vi "Scope_5160.vi"() -> ()   [LabVIEW 2013]
uses:
  <vilib>/rvi/interface/nirviReadWriteControl/nirviReadWriteControl.xnode
  <vilib>/rvi/errors/niLvFpgaAdjustHostInterfaceError.vi
  <vilib>/rvi/interface/nirviCloseFPGA/nirviCloseFPGA.xnode
  FPGA/DataMode.ctl
  NiFpgaLv.dll
  <vilib>/Utility/error.llb/Error Cluster From Error Code.vi
  <vilib>/rvi/interface/Simulation/niFpgaSimulationCallBeginRW.vi
  Host/Utilities/Ticker/Ticker.lvclass
  Host/Scope/controls/ScopeMode.ctl
  <vilib>/rvi/interface/nirviOpenFPGA/nirviOpenFPGA.xnode
  Host/Config/5160FPGAref.ctl
  Host/Scope/P2P streaming/trigger_source.ctl
  <vilib>/FPGAPlugInAG/Dynamic/niLvFpga_Close_Dynamic.vi
  FPGA Bitfiles/mixer_FPGATarget_FPGAmain5160_6pHC8ZmJ734.lvbitx
  <vilib>/FPGAPlugInAG/PXIe-7975R/niLvFpga_Open_PXIe-7975R.vi
  <vilib>/rvi/interface/common/dynamic/niFpgaDynamicAddResources.vi
  Host/Config/FPGAref.ctl
  <vilib>/userdefined/High Color/nirio_resource_hc.ctl
  <vilib>/Analysis/4window.llb/windowTd.ctl
  <vilib>/Analysis/NI_AALPro.lvlib
  Host/Scope/controls/power_spectrum_unit.ctl
panel:
  out "stop 2":bool
  out "num data 2nd loop":u32
  out "timeout counter":i32
  out "num read":u32
  out "num to clock fifo":u32
  out "error out":errorcluster
  out "P2P overflow":bool
  in  "Trigger":T1
  in  "Zoom freq X":bool
  in  "Zoom freq Y":bool
  in  "Zoom time Y":bool
  in  "Zoom time X":bool
  in  "Ch3":bool
  in  "Ch2":bool
  in  "Ch3 Q":bool
  in  "Ch3 I":bool
  in  "Ch2 Q":bool
  in  "Ch2 I":bool
  in  "input impedance":u32(ring) caption="Input Impedance" items=["1 mega ohm"=0, "50 ohms"=2]
  in  "SCOPE Resource":refnum<k15>="Dev1" caption="NI-Scope Resource"
  in  "Unit":T2
  in  "Window":T3=1 items=["Rectangle"=0, "Hanning"=1, "Hamming"=2, "Blackman-Harris"=3, "Exact Blackman"=4, "Blackman"=5, "Flat Top"=6, "4 Term B-Harris "=7, "7 Term B-Harris"=8, "Low Sidelobe"=9, "Blackman Nuttall"=11, "Triangle"=30, "Bartlett-Hanning"=31, "Bohman"=32, "Parzen"=33, "Welch"=34, "Kaiser"=60, "Dolph-Chebyshev"=61, "Gaussian"=62]
  in  "Samples per record":u32
  in  "Phase offset (deg)":dbl
  in  "Fequency [MHz]":dbl
  in  "Mode":T4
  in  "Mixer freq [MHz]":dbl
  in  "Ch1":bool
  in  "Ch0":bool
  out "freqdata":cluster{"f0":dbl, "df":dbl, "magnitude":dbl[]}[](graph)
  out "Timedata":i16[][](graph)
  in  "Rumode":bool
  in  "Singleshot":bool
  in  "Ch1 Q":bool
  in  "Ch1 I":bool
  in  "Ch0 Q":bool
  in  "Ch0 I":bool
  out "error IO":errorcluster
  in  "stop":bool
  in  "resource name":T5="RIO0"
  out "Clocking Option Configured?":bool
  out "Configured?":bool
  # "FPGA setup"
  # "Auto Zoom"
  # "Auto Zoom"
  # "FFT"
  # "Simulated data"
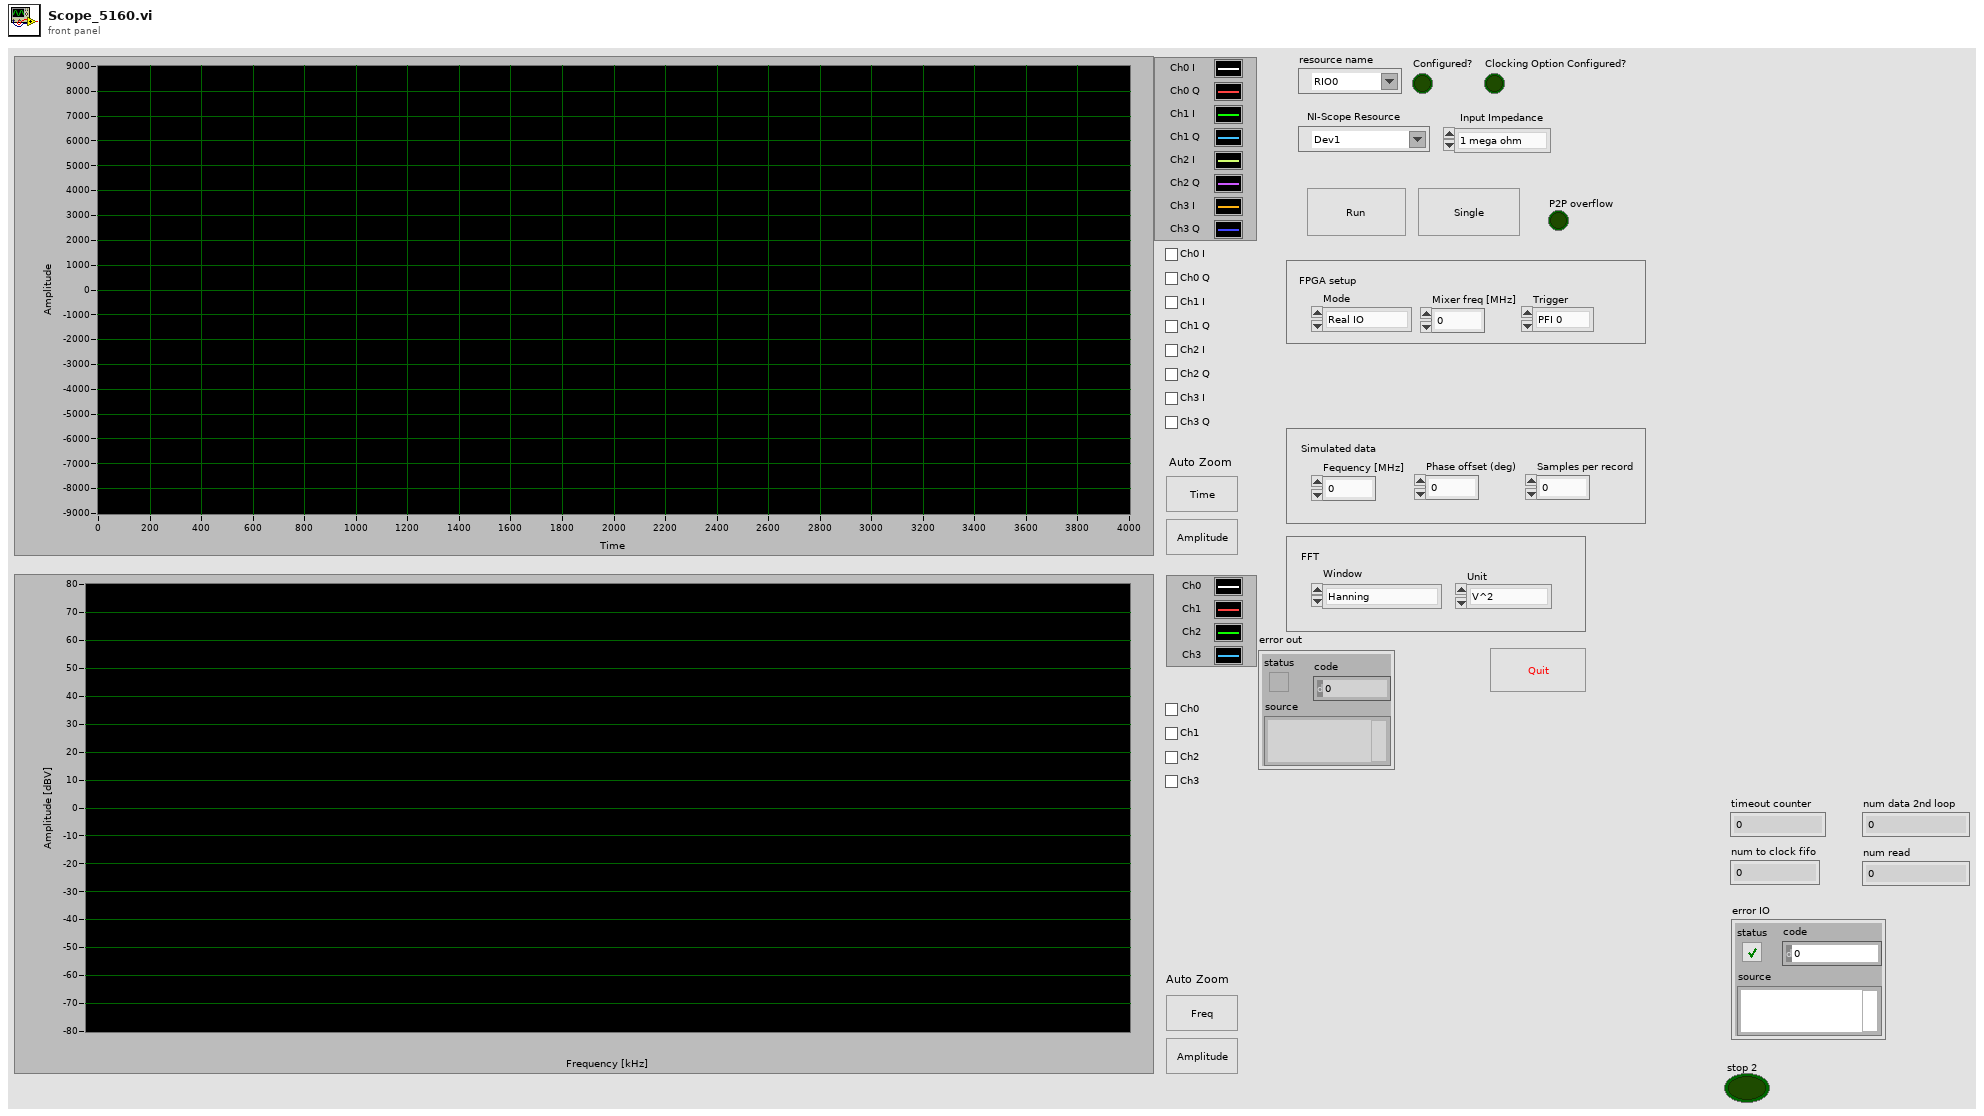
[diagram p1: front panel]
types:
  T1 = typedef "trigger_source.ctl" = enum16{"PFI 0", "PFI 1", "Software"}
  T2 = typedef "power_spectrum_unit.ctl" = enum16{"V^2", "V", "dBV"}
  T3 = typedef "NI_AALPro.lvlib/windowTd.ctl" = u32
  T4 = typedef "DataMode.ctl" = enum16{"Real IO", "Simulated"}
  T5 = typedef "nirio_resource_hc.ctl" = tag
  T6 = enum8{"Internal Clock PLL Off", "Internal Clock PLL On (REF IN)", "External Clock (CLK_IN)", "Internal Clock PLL On (IoModSyncClk)"}
  T7 = typedef "FPGAref.ctl" = refnum<k20>
  T8 = typedef "scope_params.ctl" = cluster{"scope mode":T9, "ticker":refnum<class "Ticker.lvclass">, "samples per simulated":u32, "FPGA ref":T7, "P2P params":T10, "data mode":T4}
  T9 = typedef "ScopeMode.ctl" = enum16{"Stopped", "Single", "Running"}
  T10 = typedef "P2P params.ctl" = cluster{"instrument handle":refnum<k15>, "stream session":refnum<k20>, "scale":cluster{"offset":dbl, "gain":dbl, "reserved 1":dbl, "reserved 2":dbl}, "actual sample rate":dbl, "Trigger":T1, "SCOPE Resource":refnum<k15>, "input impedance":u32}
  T11 = typedef "5160FPGAref.ctl" = refnum<k20>
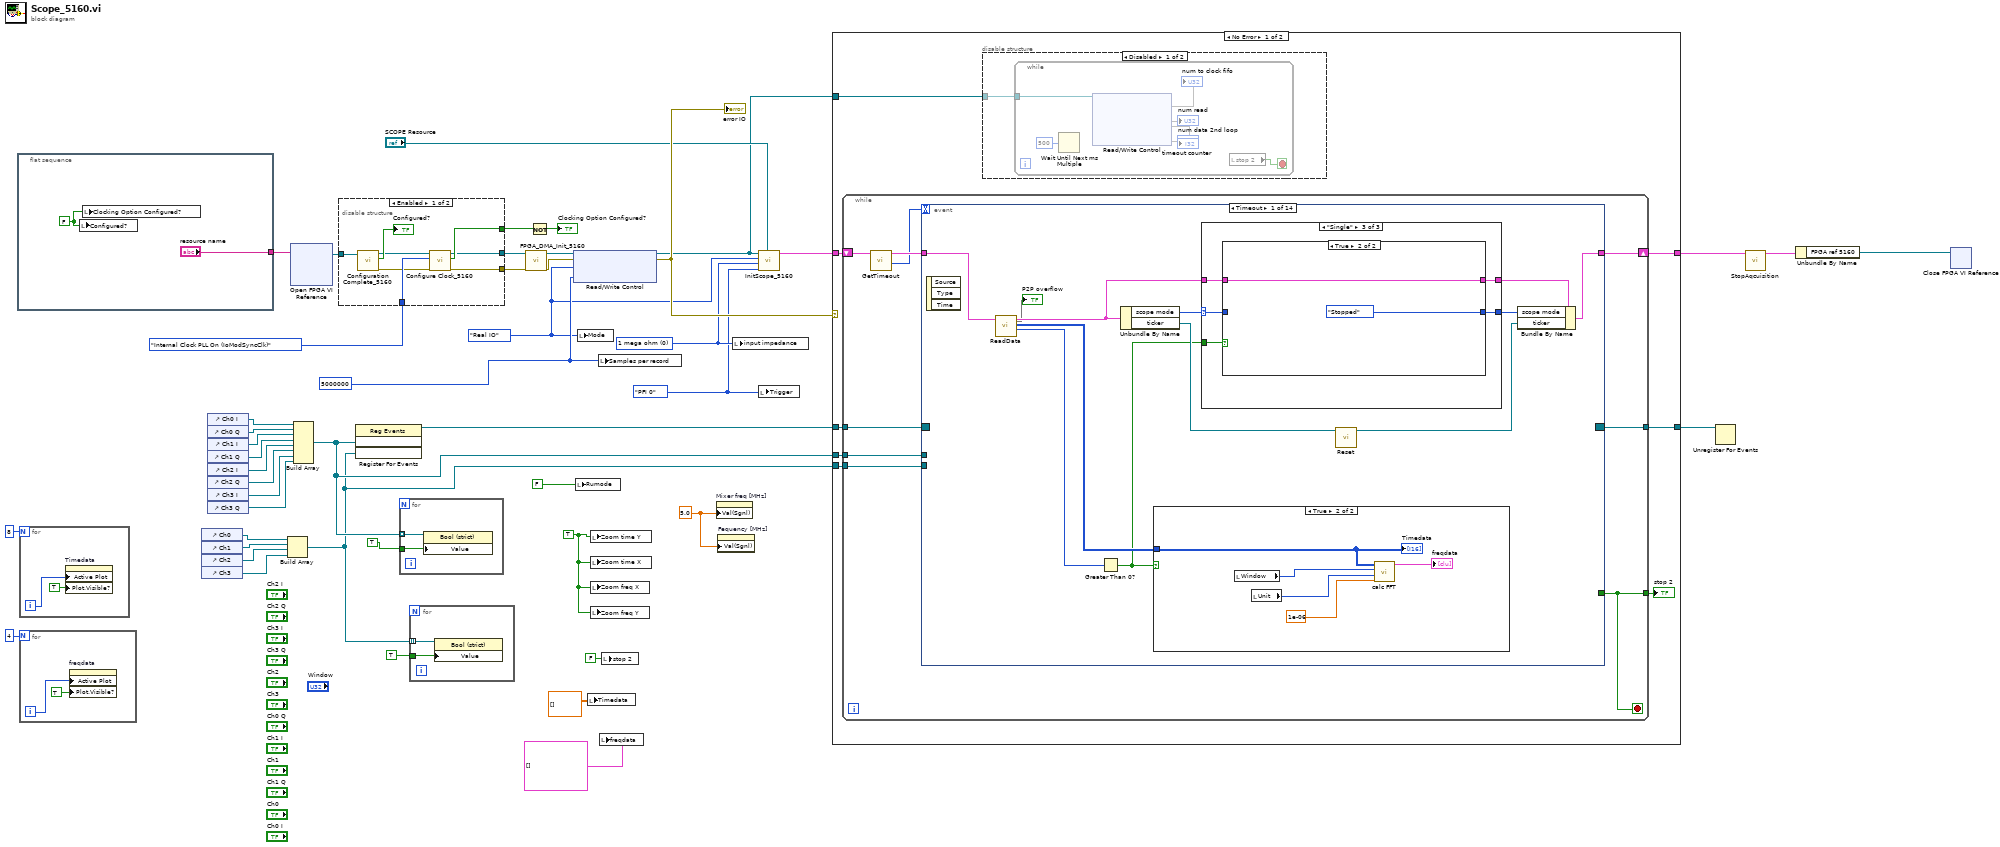
[diagram p0: block diagram]
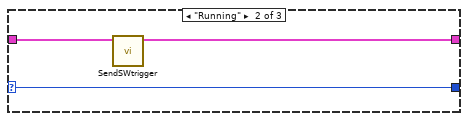
[diagram p6: hidden frame]
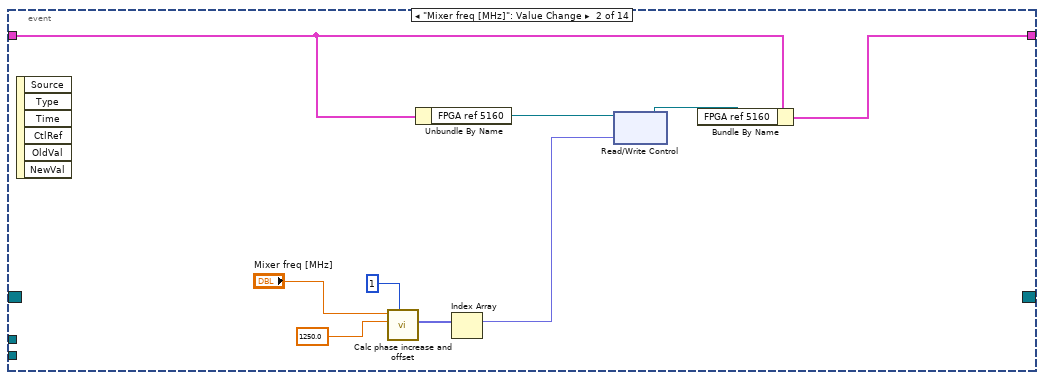
[diagram p8: hidden frame]
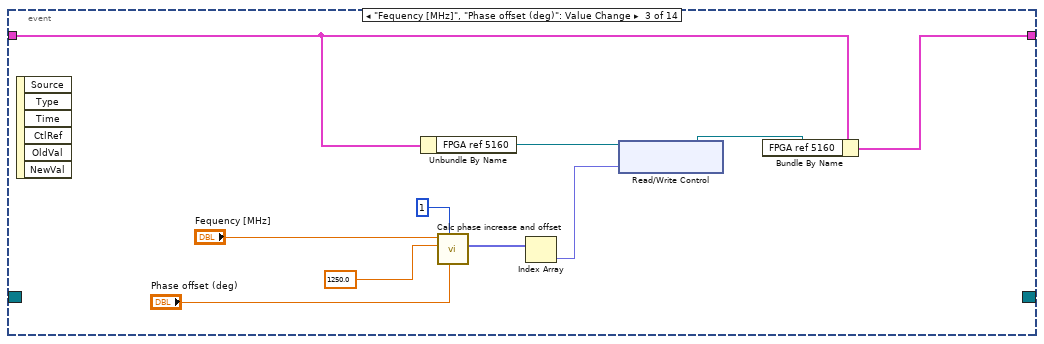
[diagram p9: hidden frame]
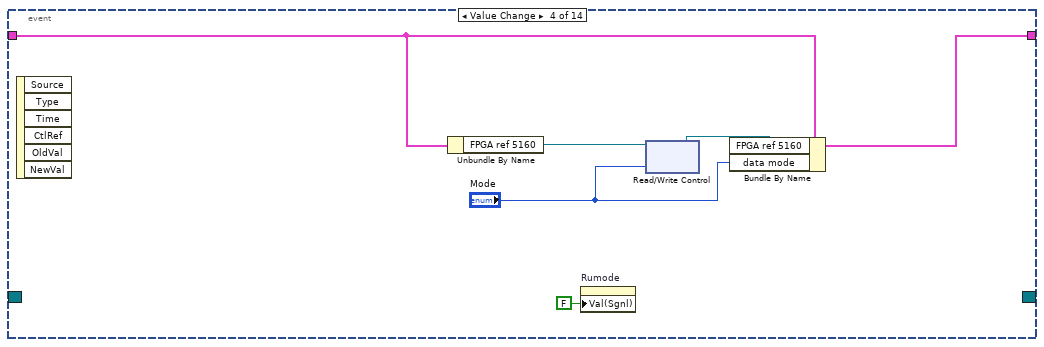
[diagram p10: hidden frame]
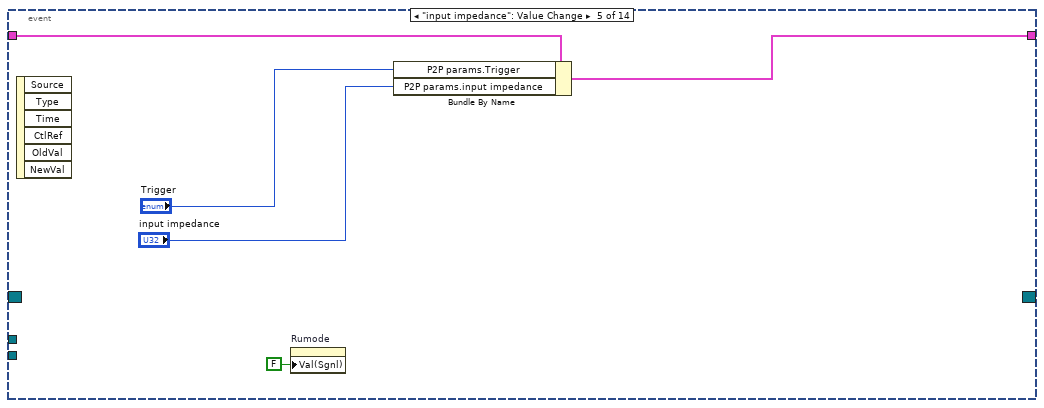
[diagram p11: hidden frame]
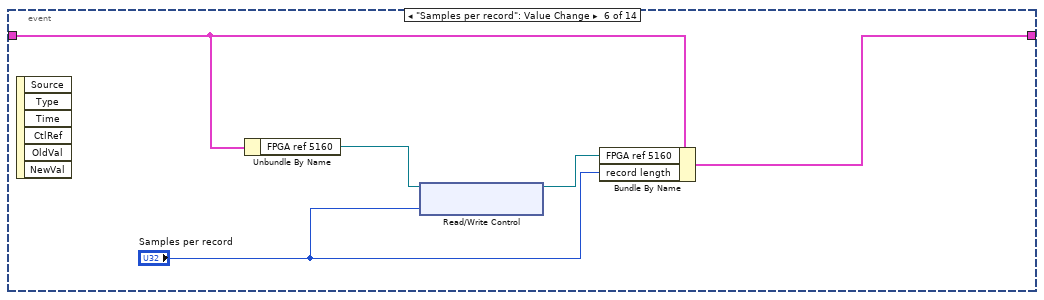
[diagram p12: hidden frame]
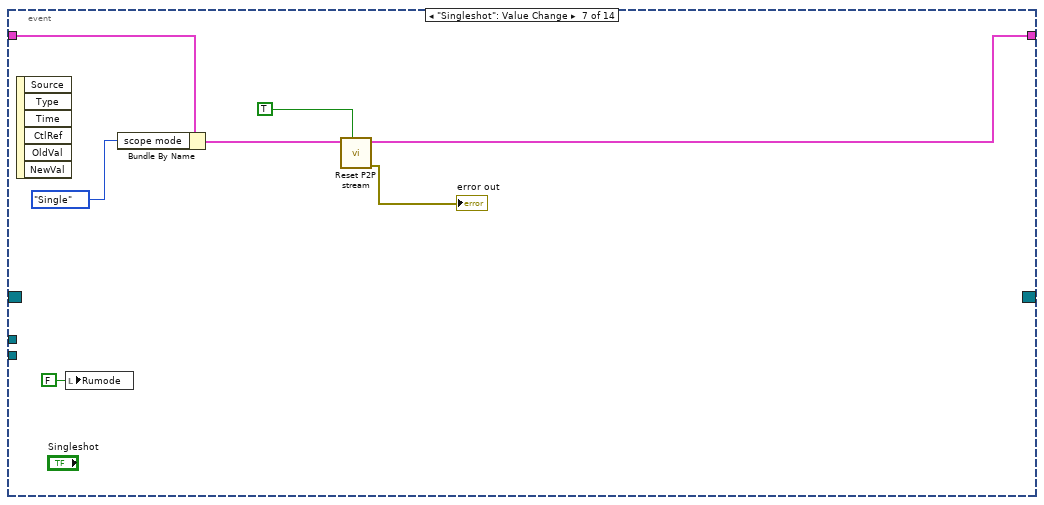
[diagram p13: hidden frame]
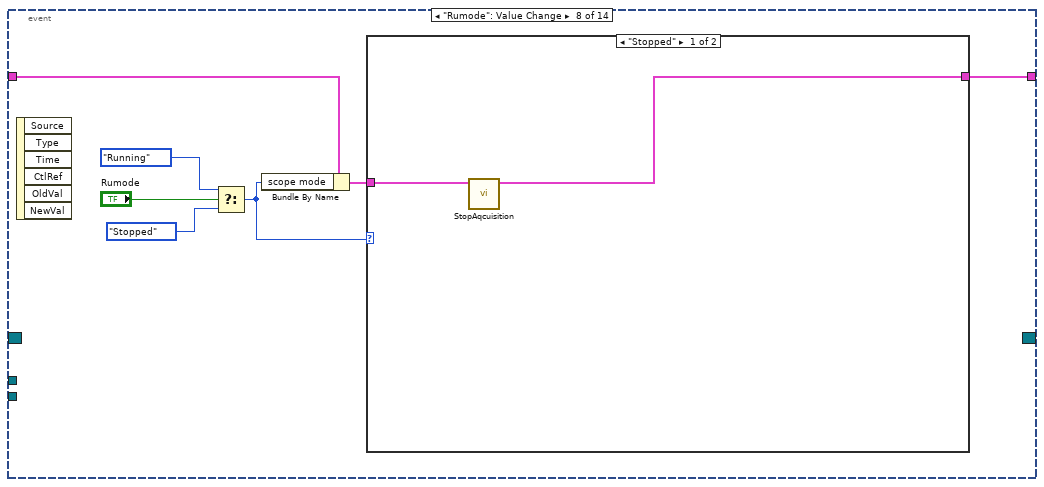
[diagram p14: hidden frame]
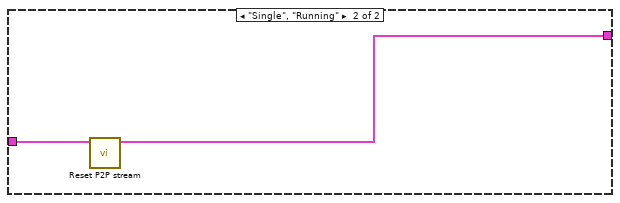
[diagram p15: hidden frame]
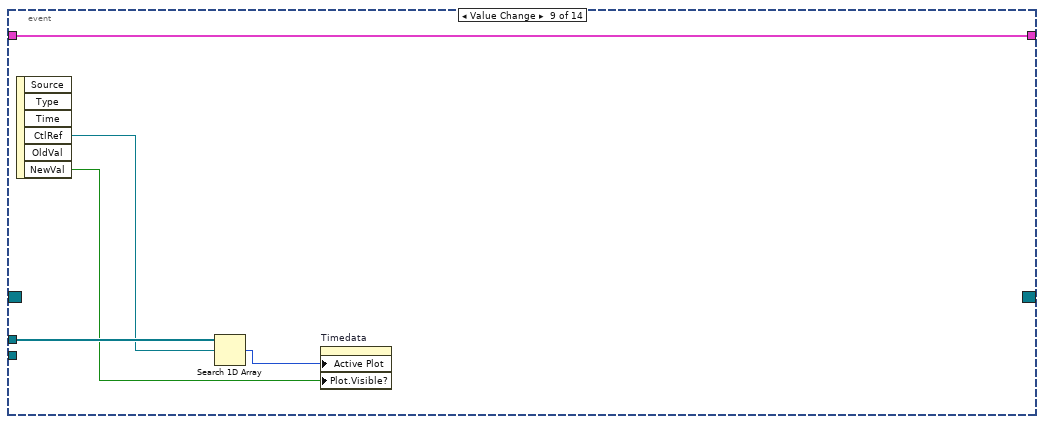
[diagram p16: hidden frame]
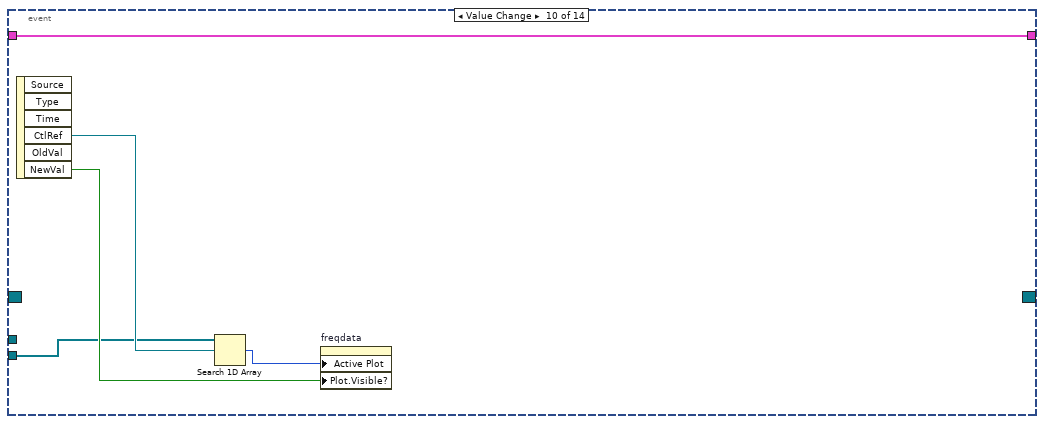
[diagram p17: hidden frame]
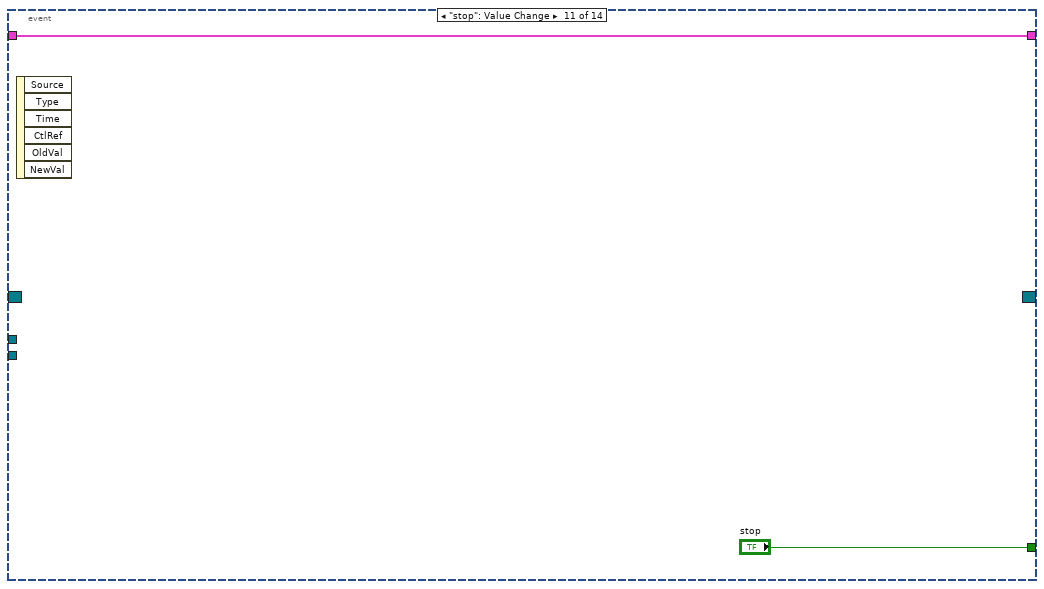
[diagram p18: hidden frame]
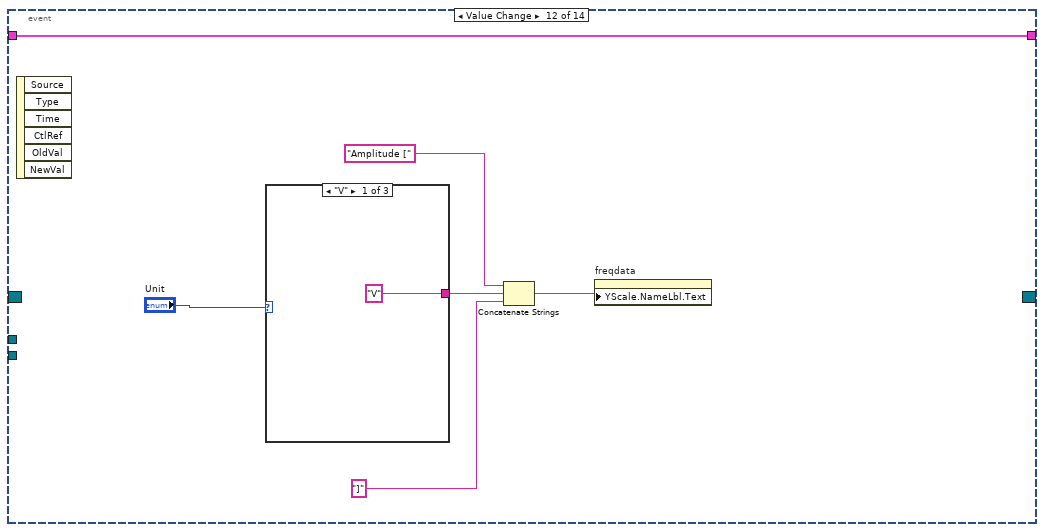
[diagram p19: hidden frame]
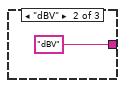
[diagram p20: hidden frame]
diagram:
  w4 = u32 0 items=["1 mega ohm"=0, "50 ohms"=2] ("input impedance")
  w3 = trigger_source."PFI 0" ("Trigger")
  w12 = TRUE ("Rumode")
  w5 = DataMode."Real IO" ("Mode")
  w7 = u32 5000000 ("Samples to aqcuire")
  w41 = 5.0 ("Mixer requency [MHz]")
  n1 = flat-sequence {
    tunnel: ["resource name"] -> w13
    frame #0 {
      w47 = FALSE ("Trigger Acquisition")
      n2 = local write "Configured?"(w47) -> ()
      n3 = local write "Clocking Option Configured?"(w47) -> ()
    }
  }
  n4 = for {
    N: 8 -> [_]
    i -> [w50]
    n5 = property on="Timedata" class="WFGraph (strict)"("Active Plot"=w50, "Plot.Visible?"=TRUE ("Plot.Visible")) -> ()  [unwired: 2 in, 2 out]
  }
  n6 = for {
    N: 4 -> [_]
    i -> [w51]
    n7 = property on="freqdata" class="WFGraph (strict)"("Active Plot"=w51, "Plot.Visible?"=TRUE ("Plot.Visible")) -> ()  [unwired: 2 in, 2 out]
  }
  n8 = control-ref of="Ch0"() -> (w26:refnum<vi>)
  n9 = control-ref of="Ch1"() -> (w25:refnum<vi>)
  n10 = control-ref of="Ch2"() -> (w24:refnum<vi>)
  n11 = control-ref of="Ch3"() -> (w23:refnum<vi>)
  n12 = control-ref of="Ch0 I"() -> (w37:refnum<vi>)
  n13 = control-ref of="Ch0 Q"() -> (w36:refnum<vi>)
  n14 = control-ref of="Ch1 I"() -> (w35:refnum<vi>)
  n15 = control-ref of="Ch1 Q"() -> (w34:refnum<vi>)
  n16 = control-ref of="Ch2 I"() -> (w33:refnum<vi>)
  n17 = control-ref of="Ch2 Q"() -> (w32:refnum<vi>)
  n18 = control-ref of="Ch3 I"() -> (w31:refnum<vi>)
  n19 = control-ref of="Ch3 Q"() -> (w30:refnum<vi>)
  n20 = Build Array(w26, w25, w24, w23) -> (w20:refnum<vi>[])
  n21 = xnode "Open FPGA VI Reference"("resource name"=w13) -> ("FPGA VI Reference Out"=w10:refnum<k20>)  [unwired: 1 in, 1 out]
  n22 = Build Array(w37, w36, w35, w34, w33, w32, w31, w30) -> (w21:refnum<vi>[])
  n23 = disable-structure shown="Enabled" {
    disable-tunnel: [w59 _] -> w18
    disable-tunnel: T6."Internal Clock PLL On (IoModSyncClk)" ("Clock Source") -> [w58 _]
    disable-tunnel: [w56 _] -> w15
    disable-tunnel: [w55 w61] -> w11
    disable-tunnel: w10 -> [w54 w61]
    frame Enabled {
      n24 = call "Configuration Complete_5160.vi"("FPGA VI Reference"=w54) -> ("error out"=w57:errorcluster, "Configured?"=→"Configured?":bool, "FPGA VI Reference out"=w53:refnum<k20>)  [unwired: 8 in]
      n25 = call "Configure Clock_5160.vi"("error in"=w57, "Clock Source"=w58, "FPGA VI Reference in"=w53) -> ("error out"=w56:errorcluster, "Configuration Error"=w59:bool, "FPGA VI Reference Out"=w55:refnum<k20>)  [unwired: 6 in]
    }
    frame Disabled {
    }
  }
  n26 = register-events(w21, w20) -> (reference out=w29:refnum<event-registration>)  [unwired: 2 in, 1 out]
  n27 = for {
    tunnel: w21 -> [w63] mode=indexing
    tunnel: TRUE ("Rumode") -> [w62]
    n28 = property class="Bool (strict)"(reference=w63, "Value"=w62) -> ()  [unwired: 1 in, 2 out]
  }
  n29 = for {
    tunnel: w20 -> [w65] mode=indexing
    tunnel: TRUE ("Rumode") -> [w64]
    n30 = property class="Bool (strict)"(reference=w65, "Value"=w64) -> ()  [unwired: 1 in, 2 out]
  }
  n31 = call "FPGA_DMA_Init_5160.vi"("error in (no error)"=w15, "FPGA VI Reference"=w11) -> ("error out"=w14:errorcluster, "FPGA VI Reference out"=w16:T7)  [unwired: 7 in, 1 out]
  n32 = Not(x=w18) -> (.not. x?=→"Clocking Option Configured?":bool)
  n33 = xnode "Read/Write Control"("FPGA VI Reference In"=w16, "error in"=w14, "Mode"=w5, "Samples Per Trigger"=w7) -> ("FPGA VI Reference Out"=w2:T7, "error out"=w44:errorcluster)
  "error IO" <- w44
  n34 = local write "Rumode"(FALSE ("Rumode")) -> ()
  n35 = local write "Mode"(w5) -> ()
  n36 = local write "Timedata"(dbl[][] [] ("Timedata")) -> ()
  n37 = local write "Zoom time Y"(w12) -> ()
  n38 = local write "Zoom time X"(w12) -> ()
  n39 = local write "Zoom freq X"(w12) -> ()
  n40 = local write "Zoom freq Y"(w12) -> ()
  n41 = local write "Samples per record"(w7) -> ()
  n42 = local write "freqdata"(cluster{"f0":dbl, "df":dbl, "magnitude":dbl[]}[] [] ("freqdata")) -> ()
  n43 = local write "stop 2"(FALSE ("stop 2")) -> ()
  n44 = property on="Mixer freq [MHz]" class="DigNum (strict)"("Val(Sgnl)"=w41) -> ()  [unwired: 2 in, 2 out]
  n45 = property on="Fequency [MHz]" class="DigNum (strict)"("Val(Sgnl)"=w41) -> ()  [unwired: 2 in, 2 out]
  n46 = local write "input impedance"(w4) -> ()
  n47 = call "InitScope_5160.vi"("SCOPE Resource"="SCOPE Resource", "error in"=w3, "input impedance"=w4, "data mode"=w5, "FPGA ref"=w2) -> ("scope params"=w46:T8)  [unwired: 5 in, 1 out]
  n48 = local write "Trigger"(w3) -> ()
  n49 = case shown="No Error" w44 {
    tunnel: w46 -> [w73 w205]
    tunnel: [w72 w205] -> w9
    tunnel: w29 -> [w71 w204]
    tunnel: [w70 w204] -> w28
    tunnel: w21 -> [w69 _]
    tunnel: w20 -> [w68 _]
    tunnel: w2 -> [w66 _]
    frame No Error {
      n50 = while {
        shift-right: [w90] -> w72
        shift-left: w73 -> [w89]
        tunnel: w71 -> [w86]
        tunnel: [w85] -> w70
        tunnel: w69 -> [w84]
        tunnel: w68 -> [w83]
        tunnel: [w82] -> w67
        stop <- w82 stop-if-true
        n51 = call "GetTimeout.vi"("scope in"=w89) -> ("Time left"=w87:i32, "scope out"=w88:T8)  [unwired: 9 in]
        n52 = event shown="[0] Timeout" {
          selector: w86 -> [_ _ _ _ _ _ _ _ _ _ _ _ _ _]
          dyn-events: [_ _ _ _ _ _ _ _ _ _ _ _ _ _] -> w85
          timeout: w87 -> [_ _ _ _ _ _ _ _ _ _ _ _ _ _]
          tunnel: [_ _ _ _ _ _ _ _ _ _ "stop" _ _ _] -> w82
          tunnel: w88 -> [w97 w125 w136 w144 w150 w153 w161 w166 w179 w184 w185 w192 w199 w203]
          tunnel: [w100 w123 w135 w143 w147 w152 w158 w164 w179 w184 w185 w192 w199 w203] -> w90
          tunnel: w84 -> [_ _ _ _ _ _ _ _ w178 _ _ _ _ _]
          tunnel: w83 -> [_ _ _ _ _ _ _ _ _ w180 _ _ _ _]
          event Timeout {
            n53 = event-data() -> ()  [unwired: 1 in, 3 out]
            n54 = call "ReadData.vi"("scope params"=w97) -> ("Num elements"=w94:i32, "data"=w93:i16[][], "scope params out"=w96:T8, 5:→"P2P overflow")  [unwired: 7 in]
            n55 = Greater Than 0?(x=w94) -> (x > 0?=w91:bool)
            n56 = Unbundle By Name(w96) -> ("scope mode"=w99:T9, "ticker"=w102:refnum<class "Ticker.lvclass">)
            n57 = case shown="True" w91 {
              tunnel: w93 -> [_ w103]
              frame False {
              }
              frame True {
                n58 = local read "Window"() -> (w106:T3)
                n59 = local read "Unit"() -> (w105:T2)
                n60 = call "calc FFT.vi"("dt"=1e-06, "Unit"=w105, "Window"=w106, "data"=w103) -> ("Power Spectrum / PSD"=→"freqdata":cluster{"f0":dbl, "df":dbl, "magnitude":dbl[]}[])  [unwired: 7 in]
                "Timedata" <- w103
              }
            }
            n61 = case shown="\"Single\"" w99 {
              selector: w99 -> [w109 w112 w113]
              tunnel: [w109 w112 w117] -> w98
              tunnel: w96 -> [w108 w111 w116]
              tunnel: [w108 w110 w115] -> w95
              tunnel: w91 -> [_ _ w114]
              frame "Stopped" {
              }
              frame "Running" {
                n62 = call "SendSWtrigger.vi"("scope in"=w111) -> ("scope out"=w110:T8)  [unwired: 9 in, 1 out]
              }
              frame "Single" {
                n63 = case shown="True" w114 {
                  tunnel: [w118 ScopeMode."Stopped" ("scope mode")] -> w117
                  tunnel: w116 -> [w119 w120]
                  tunnel: [w119 w120] -> w115
                  tunnel: w113 -> [w118 _]
                  frame False {
                  }
                  frame True {
                  }
                }
              }
            }
            n64 = call "Reset.vi"("Ticker in"=w102) -> ("Ticker out"=w101:refnum<class "Ticker.lvclass">)  [unwired: 9 in, 1 out]
            n65 = Bundle By Name(cluster=w95, "scope mode"=w98, "ticker"=w101) -> (w100:T8)
          }
          event "Mixer freq [MHz]": Value Change {
            n66 = event-data() -> ()  [unwired: 1 in, 6 out]
            n67 = call "Calc phase increase and offset.vi"("# of DDS"=1, "fclk (MHz)"=1250.0 ("fclk (800MHz)"), "f_generated (MHz)"="Mixer freq [MHz]") -> ("Phase out"=w128:fxp<+,64,64>[])  [unwired: 6 in, 2 out]
            n68 = Unbundle By Name(w125) -> ("FPGA ref 5160"=w126:T11)
            n69 = Index Array(array=w128) -> (element=w122:fxp<+,64,64>)  [unwired: 1 in]
            n70 = xnode "Read/Write Control"("FPGA VI Reference In"=w126, "phase"=w122) -> ("FPGA VI Reference Out"=w124:T11)  [unwired: 1 in, 1 out]
            n71 = Bundle By Name(cluster=w125, "FPGA ref 5160"=w124) -> (w123:T8)
          }
          event "Fequency [MHz]", "Phase offset (deg)": Value Change {
            n72 = event-data() -> ()  [unwired: 1 in, 6 out]
            n73 = Unbundle By Name(w136) -> ("FPGA ref 5160"=w138:T11)
            n74 = call "Calc phase increase and offset.vi"("Phase offset (deg)"="Phase offset (deg)", "# of DDS"=1, "fclk (MHz)"=1250.0 ("fclk (800MHz)"), "f_generated (MHz)"="Fequency [MHz]") -> ("Phase out"=w134:fxp<+,64,64>[])  [unwired: 5 in, 2 out]
            n75 = Index Array(array=w134) -> (element=w131:fxp<+,64,64>)  [unwired: 1 in]
            n76 = xnode "Read/Write Control"("FPGA VI Reference In"=w138, "simulated phase"=w131) -> ("FPGA VI Reference Out"=w137:T11)  [unwired: 1 in, 1 out]
            n77 = Bundle By Name(cluster=w136, "FPGA ref 5160"=w137) -> (w135:T8)
          }
          event Value Change {
            n78 = event-data() -> ()  [unwired: 1 in, 6 out]
            n79 = Unbundle By Name(w144) -> ("FPGA ref 5160"=w146:T11)
            n80 = property on="Rumode" class="Bool (strict)"("Val(Sgnl)"=FALSE ("Value (Signaling)")) -> ()  [unwired: 2 in, 2 out]
            n81 = xnode "Read/Write Control"("FPGA VI Reference In"=w146, "Mode"="Mode") -> ("FPGA VI Reference Out"=w145:T11)  [unwired: 1 in, 1 out]
            n82 = Bundle By Name(cluster=w144, "FPGA ref 5160"=w145, "data mode"="Mode") -> (w143:T8)
          }
          event "input impedance": Value Change {
            n83 = event-data() -> ()  [unwired: 1 in, 6 out]
            n84 = property on="Rumode" class="Bool (strict)"("Val(Sgnl)"=FALSE ("Value (Signaling)")) -> ()  [unwired: 2 in, 2 out]
            n85 = Bundle By Name(cluster=w150, "P2P params.Trigger"="Trigger", "P2P params.input impedance"="input impedance") -> (w147:T8)
          }
          event "Samples per record": Value Change {
            n86 = event-data() -> ()  [unwired: 1 in, 6 out]
            n87 = Unbundle By Name(w153) -> ("FPGA ref 5160"=w156:T11)
            n88 = xnode "Read/Write Control"("FPGA VI Reference In"=w156, "Samples Per Trigger"="Samples per record") -> ("FPGA VI Reference Out"=w155:T11)  [unwired: 1 in, 1 out]
            n89 = Bundle By Name(cluster=w153, "FPGA ref 5160"=w155, "record length"="Samples per record") -> (w152:T8)
          }
          event "Singleshot": Value Change {
            n90 = event-data() -> ()  [unwired: 1 in, 6 out]
            n91 = local write "Rumode"(FALSE ("Rumode")) -> ()
            n92 = Bundle By Name(cluster=w161, "scope mode"=ScopeMode."Single") -> (w160:T8)
            n93 = call "Reset P2P stream.vi"("single shot"=TRUE, "scope params"=w160) -> ("error out"=→"error out":errorcluster, "scope params out"=w158:T8)  [unwired: 8 in]
          }
          event "Rumode": Value Change {
            n94 = event-data() -> ()  [unwired: 1 in, 6 out]
            n95 = Select(t=ScopeMode."Running" ("scope mode"), s="Rumode", f=ScopeMode."Stopped" ("scope mode")) -> (s? t:f=w165:T9)
            n96 = Bundle By Name(cluster=w166, "scope mode"=w165) -> (w167:T8)
            n97 = case shown="\"Stopped\"" w165 {
              tunnel: w167 -> [w172 w174]
              tunnel: [w171 w173] -> w164
              frame "Stopped" {
                n98 = call "StopAqcuisition.vi"("scope in"=w172) -> ("scope out"=w171:T8)  [unwired: 9 in, 1 out]
              }
              frame "Single", "Running" {
                n99 = call "Reset P2P stream.vi"("scope params"=w174) -> ("scope params out"=w173:T8)  [unwired: 9 in, 1 out]
              }
            }
          }
          event Value Change {
            n100 = event-data() -> ("CtlRef"=w177:refnum<vi>, "NewVal"=w175:bool)  [unwired: 1 in, 4 out]
            n101 = Search 1D Array(1D array=w178, element=w177) -> (index of element=w176:i32)  [unwired: 1 in]
            n102 = property on="Timedata" class="WFGraph (strict)"("Active Plot"=w176, "Plot.Visible?"=w175) -> ()  [unwired: 2 in, 2 out]
          }
          event Value Change {
            n103 = event-data() -> ("CtlRef"=w183:refnum<vi>, "NewVal"=w181:bool)  [unwired: 1 in, 4 out]
            n104 = Search 1D Array(1D array=w180, element=w183) -> (index of element=w182:i32)  [unwired: 1 in]
            n105 = property on="freqdata" class="WFGraph (strict)"("Active Plot"=w182, "Plot.Visible?"=w181) -> ()  [unwired: 2 in, 2 out]
          }
          event "stop": Value Change {
            n106 = event-data() -> ()  [unwired: 1 in, 6 out]
          }
          event Value Change {
            n107 = event-data() -> ()  [unwired: 1 in, 6 out]
            n108 = case shown="\"V\"" "Unit" {
              tunnel: ["V" "dBV" "V^2"] -> w189
              frame "V" {
              }
              frame "dBV" {
              }
              frame "V^2" {
              }
            }
            n109 = Concatenate Strings("Amplitude [", w189, "]") -> (w187:string)
            n110 = property on="freqdata" class="WFGraph (strict)"("YScale.NameLbl.Text"=w187) -> ()  [unwired: 2 in, 2 out]
          }
          event "Zoom time X", "Zoom time Y": Value Change {
            n111 = event-data() -> ()  [unwired: 1 in, 6 out]
            n112 = control-ref of="Timedata"() -> (w198:refnum<vi>)
            n113 = call "setZoomTool.vi"("Zoom Y"="Zoom time Y", "Zoom  X"="Zoom time X", "reference"=w198) -> ()  [unwired: 9 in]
          }
          event "Zoom freq Y", "Zoom freq X": Value Change {
            n114 = event-data() -> ()  [unwired: 1 in, 6 out]
            n115 = control-ref of="freqdata"() -> (w200:refnum<vi>)
            n116 = call "setZoomTool.vi"("Zoom Y"="Zoom freq Y", "Zoom  X"="Zoom freq X", "reference"=w200) -> ()  [unwired: 9 in]
          }
        }
      }
      "stop 2" <- w67
      n117 = disable-structure shown="Disabled" {
        disable-tunnel: w66 -> [w74 _]
        frame Disabled {
          n118 = while {
            tunnel: w74 -> [w75]
            stop <- w76 stop-if-true
            n119 = Wait Until Next ms Multiple(millisecond multiple=u32 500) -> ()  [unwired: 1 out]
            n120 = xnode "Read/Write Control"("FPGA VI Reference In"=w75) -> ("num to clock fifo"=→"num to clock fifo", "num read"=→"num read", "timeout counter"=→"timeout counter", "num data 2nd loop"=→"num data 2nd loop")  [unwired: 1 in, 2 out]
            n121 = local read "stop 2"() -> (w76:bool)
          }
        }
        frame Enabled {
        }
      }
    }
    frame Error {
    }
  }
  n122 = Unregister For Events(event registration refnum=w28) -> ()  [unwired: 1 in, 1 out]
  n123 = call "StopAqcuisition.vi"("scope in"=w9) -> ("scope out"=w8:T8)  [unwired: 9 in, 1 out]
  n124 = Unbundle By Name(w8) -> ("FPGA ref 5160"=w45:T11)
  n125 = xnode "Close FPGA VI Reference"("FPGA VI Reference In"=w45) -> ()  [unwired: 1 in, 1 out]
